vi "Remove.vi"(11 "TypedCircularBuffer in":refnum<class "RotateCircularBuffer.lvclass">) -> (1 "invalid?":bool, 2 "element":T1, 3 "TypedCircularBuffer out":refnum<class "RotateCircularBuffer.lvclass">)   [LabVIEW 2024, in "RotateCircularBuffer.lvclass"]
uses:
  RotateCircularBuffer.lvclass
  Type.ctl
  RotateCircularBuffer.lvclass/RotateCircularBuffer.ctl
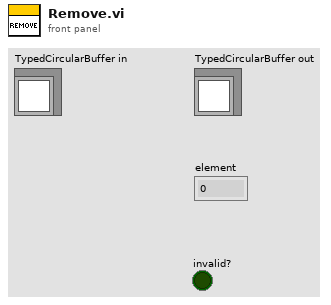
[diagram p1: front panel]
types:
  T1 = typedef "RotateCircularBuffer.lvclass/Type.ctl" = u8
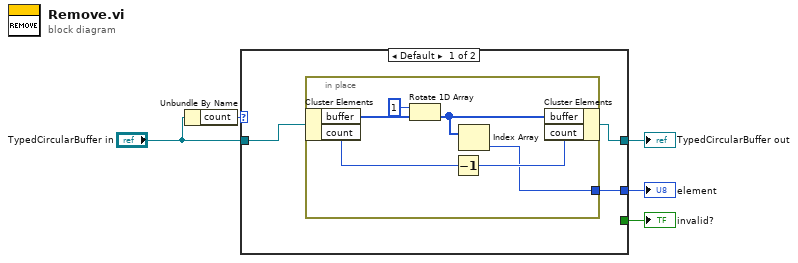
[diagram p0: block diagram]
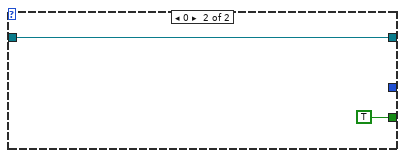
[diagram p2: hidden frame]
diagram:
  n1 = Unbundle By Name("TypedCircularBuffer in") -> ("count"=w3:u32)
  n2 = case shown="Default" w3 {
    tunnel: "TypedCircularBuffer in" -> [w8 w16]
    tunnel: [w7 w16] -> w4
    tunnel: [w6 _] -> w2
    tunnel: [_ TRUE] -> w1
    frame Default {
      n3 = in-place {
        in-place-border: [w11] -> w6
        n4 = in-place-cluster #1(w8) -> ("buffer"=w12:T1[], "count"=w14:u32)
        n5 = Rotate 1D Array(1:w12, 2:1 ("n")) -> (0:w9:T1[])
        n6 = Decrement(x=w14) -> (x-1=w13:u32)
        n7 = Index Array(array=w9) -> (element=w11:T1)  [unwired: 1 in]
        n8 = in-place-cluster #1("buffer"=w9, "count"=w13) -> (w7:refnum<class "RotateCircularBuffer.lvclass">)
      }
    }
    frame 0 {
    }
  }
  "TypedCircularBuffer out" <- w4
  "element" <- w2
  "invalid?" <- w1
